vi "Chi-Squared (Non-Central) PDF.vi"(9 "d":dbl, 10 "k":i32=1, 11 "x":dbl=1.0) -> (0 "error":i32, 3 "pdf(x)":dbl=0.24197072451914334)   [LabVIEW 2014, in "NI_Gmath.lvlib"]
doc: "Computes the continuous probability density function (PDF) of various distributions. You must manually select the polymorphic instance to use."
uses:
  NI_Gmath.lvlib
  st_error_code.ctl
  Gamma Function.vi
panel:
  # "Chi-Squared (Non-Central) PDF"
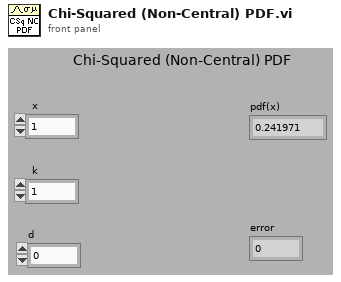
[diagram p1: front panel]
types:
  T1 = typedef "NI_Gmath.lvlib/st_error_code.ctl" = i32
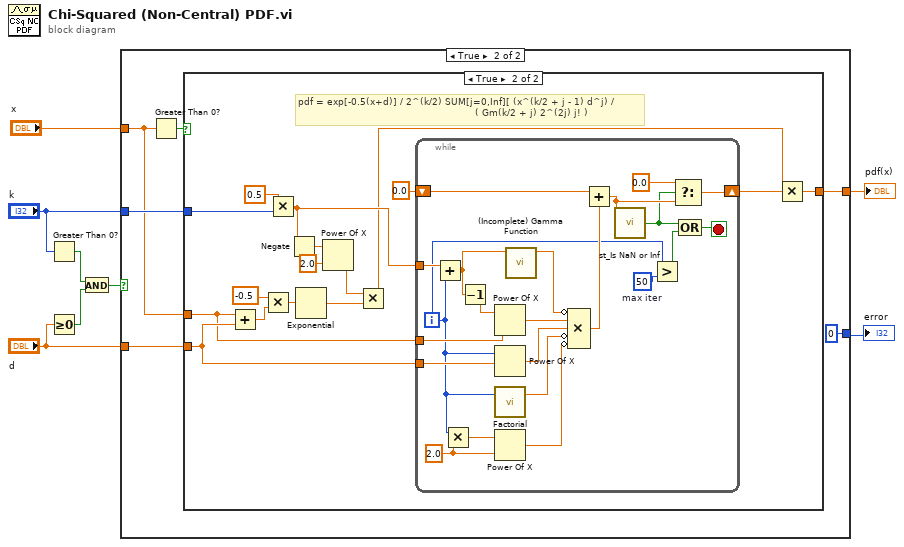
[diagram p0: block diagram]
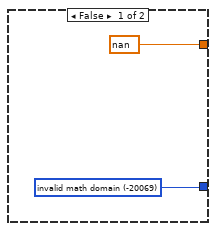
[diagram p2: hidden frame]
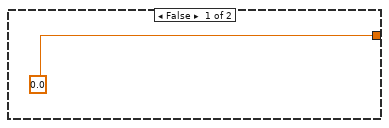
[diagram p3: hidden frame]
diagram:
  n1 = Greater Than 0?(x="k") -> (x > 0?=w4:bool)
  n2 = Greater Or Equal To 0?(x="d") -> (x >= 0?=w2:bool)
  n3 = And(x=w4, y=w2) -> (x .and. y?=w5:bool)
  n4 = case shown="True" w5 {
    tunnel: [w9 0 ("invalid math domain")] -> w8
    tunnel: [nan w15] -> w7
    tunnel: "x" -> [_ w13]
    tunnel: "k" -> [_ w14]
    tunnel: "d" -> [_ w11]
    frame False {
      w9 = T1 -20069 items=["invalid math domain"=-20069, "Fourier interpolation size m >= n"=-20070, "empty array"=-20003] ("stat interp error code")
    }
    frame True {
      n5 = Greater Than 0?(x=w13) -> (x > 0?=w12:bool)
      n6 = case shown="True" w12 {
        tunnel: [0.0 w19] -> w15
        tunnel: w13 -> [_ w22]
        tunnel: w14 -> [_ w33]
        tunnel: w11 -> [_ w23]
        frame False {
        }
        frame True {
          # "pdf = exp[-0.5(x+d)] / 2^(k/2) SUM[j=0,Inf][ (x^(k/2 + j - 1) d^j) /\n                                                           ( Gm(k/2 + j) 2^(2j) j! )"
          n7 = Add(x=w22, y=w23) -> (x+y=w32:dbl)
          n8 = Multiply(x=-0.5, y=w32) -> (x*y=w30:dbl)
          n9 = Multiply(x=0.5, y=w33) -> (x*y=w21:dbl)
          n10 = Negate(x=w21) -> (-x=w26:dbl)
          n11 = Exponential(1:w30) -> (0:w28:dbl)
          n12 = Power Of X(1:2.0 ("x"), 2:w26) -> (0:w25:dbl)
          n13 = Multiply(x=w25, y=w28) -> (x*y=w18:dbl)
          n14 = while {
            shift-right: [w40] -> w20
            shift-left: 0.0 ("x") -> [w43]
            tunnel: w22 -> [w55]
            tunnel: w21 -> [w54]
            tunnel: w23 -> [w53]
            i -> [w34]
            stop <- w37 stop-if-true
            w38 = 50  # max iter
            w50 = 2.0 ("x")
            n15 = Add(x=w54, y=w34) -> (x+y=w47:dbl)
            n16 = Multiply(x=w34, y=w50) -> (x*y=w49:dbl)
            n17 = Decrement(x=w47) -> (x-1=w48:dbl)
            n18 = Power Of X(1:w55, 2:w48) -> (0:w51:dbl)
            n19 = Power Of X(1:w53, 2:w34) -> (0:w52:dbl)
            n20 = call "Factorial.vi"("n"=w34) -> ("n!"=w45:dbl)  [unwired: 2 in]
            n21 = Power Of X(1:w50, 2:w49) -> (0:w44:dbl)
            n22 = call-poly "(Incomplete) Gamma Function.vi"("x"=w47) -> ("g(x)"=w46:dbl)  [unwired: 10 in]
            n23 = Compound Arithmetic op=MULTIPLY(invert w46, w51, w52, invert w45, invert w44) -> (w39:dbl)
            n24 = Add(x=w43, y=w39) -> (x+y=w41:dbl)
            n25 = call "st_Is NaN or Inf.vi"("x"=w41) -> ("isNaN(x) || isInf(x)"=w36:bool)  [unwired: 4 in]
            n26 = Greater?(x=w34, y=w38) -> (0:w35:bool)
            n27 = Select(t=0.0, s=w36, f=w41) -> (s? t:f=w40:dbl)
            n28 = Compound Arithmetic op=OR(w36, w35) -> (w37:bool)
          }
          n29 = Multiply(x=w18, y=w20) -> (x*y=w19:dbl)
        }
      }
    }
  }
  "pdf(x)" <- w7
  "error" <- w8
